vi "Start Arrival Time Counters TIO.vi"(7 "Save Data":bool, 8 "error in":errorcluster) -> (0 "error out":errorcluster, 1 "Column Definitions":T2(array[cluster]) {"Offset" format="%.2f"; "Resolution" format="%.2f"}, 2 "Buffer":i32[][](array[numeric]), 3 "Arrival Time Clusters":T3(array[cluster]), 5 "Temp File Definition":T1)   [LabVIEW 2009]
uses:
  Acquisition Settings.vi
panel:
  in  "Arrival Time Cluster":T4 {"task ID out" format="%.0x"}
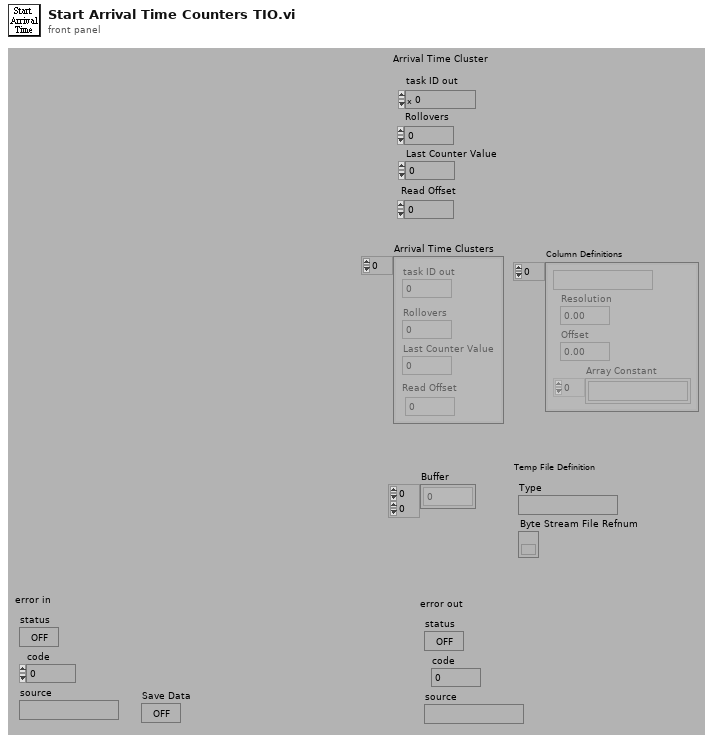
[diagram p1: front panel]
types:
  T1 = cluster{"Type":string, "Byte Stream File Refnum":refnum<file>}
  T2 = cluster{string, "Resolution":dbl, "Offset":dbl, "Array Constant":string[]}[]
  T3 = cluster{"task ID out":u32, "Rollovers":i32, "Last Counter Value":u32, "Read Offset":i32}[]
  T4 = cluster{"task ID out":u32, "Rollovers":i32, "Last Counter Value":u32, "Read Offset":i32}
  T5 = cluster{"Name":string, "Device Number":i16, "Counter Number":i16, "Line Type for Gate":u32, "Line Number for Gate":u32, "Line Type for Source":u32, "Line Number for Source":u32, "Transfer Method":u32, "Signal Routing Configuration":i16}[]
  T6 = cluster{string, dbl, "Offset":dbl, "Array Constant":string[]}
  T7 = cluster{string, "Resolution":dbl, "Offset":dbl, "Array Constant":string[]}
  T8 = cluster{"Name":string, "Signal Routing":cluster{"signal name":u16, "signal source":u16, "signal source line number":u32, "signal name line number":u32}[]}[]
  T9 = cluster{"Name":string, "Signal Routing":cluster{"signal name":u16, "signal source":u16, "signal source line number":u32, "signal name line number":u32}[]}
  T10 = cluster{"signal name":u16, "signal source":u16, "signal source line number":u32, "signal name line number":u32}[]
  T11 = cluster{string, "Offset":dbl, "Offset":dbl, string[]}
  T12 = cluster{string, "Offset":dbl, "Offset":dbl, "Array Constant":string[]}[]
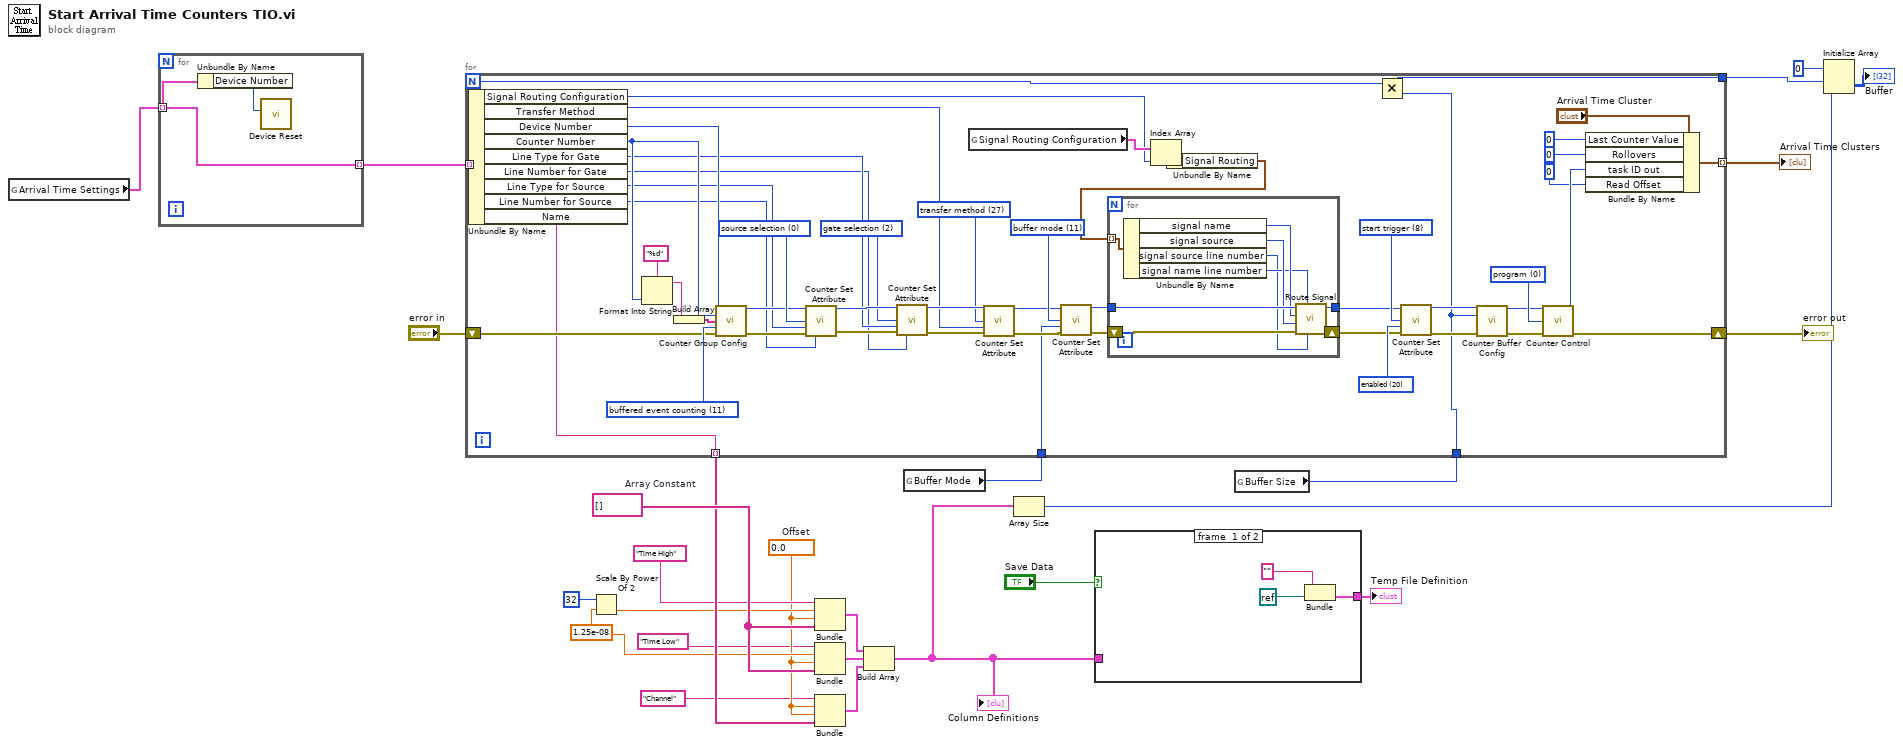
[diagram p0: block diagram]
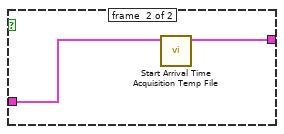
[diagram p2: hidden frame]
diagram:
  w9 = 0.0  # Offset
  w10 = 1.25e-08 ("Resolution")
  w18 = string[] []  # Array Constant
  n1 = global read "Acquisition Settings.vi" "Arrival Time Settings"() -> (w3:T5)
  n2 = for {
    tunnel: w3 -> [w28] mode=indexing
    tunnel: [w28] -> w4 mode=indexing
    n3 = Unbundle By Name(w28) -> ("Device Number"=w27:i16)
    n4 = call <vilib>:"Device Reset.vi"("device"=w27) -> ()  [unwired: 9 in, 2 out]
  }
  n5 = Scale By Power Of 2(n=32, x=w10) -> (x*2^n=w12:dbl)
  n6 = Bundle("Time High", w12, "Offset"=w9, "Array Constant"=w18) -> (w16:T6)  [unwired: 1 in]
  n7 = Bundle("Time Low", "Resolution"=w10, "Offset"=w9, "Array Constant"=w18) -> (w15:T7)  [unwired: 1 in]
  n8 = global read "Acquisition Settings.vi" "Buffer Mode"() -> (w2:u32)
  n9 = global read "Acquisition Settings.vi" "Buffer Size"() -> (w1:i32)
  n10 = for {
    N -> [w48]
    shift-right: [w60] -> w26
    shift-left: "error in" -> [w59]
    tunnel: w4 -> [w58] mode=indexing
    tunnel: [w47] -> w23
    tunnel: [w53] -> w22 mode=indexing
    tunnel: [w45] -> w17 mode=indexing
    tunnel: w2 -> [w38]
    tunnel: w1 -> [w37]
    w40 = u32 27 items=["source selection", "source polarity", "gate selection", "gate polarity", "output mode", "output polarity", "aux line selection", "aux line polarity", "start trigger", "counting synchronous", "up down", "buffer mode", "encoder type", "initial count", "pulse spec 1", "pulse spec 2", "pulse spec 3", "pulse spec 4", "auto increment", "prescale value", "Z index active", "Z index value", "Z index reload phase", "(Reserved) synchronization line", "(Reserved) synchronization method", "(Reserved) seconds", "(Reserved) precision", "transfer method", "start trigger polarity"] ("attribute ID")
    w54 = u32 20 items=["yes", "no", "positive", "negative", "high", "low", "low to high", "high to low", "default", "max timebase", "other counter gate", "other counter TC", "other counter output", "other counter source", "source", "gate", "aux line", "in start trigger", "in stop trigger", "automatic", "enabled", "count up", "count down", "hardware", "single", "double", "pulse", "toggle", "quadrature encoder X1", "quadrature encoder X2", "quadrature encoder X4", "two pulse counting", "A high B high", "A high B low", "A low B high", "A low B low", "PFI n", "RTSI n", "timebase n"] ("attribute value type")
    w55 = u32 8 items=["source selection", "source polarity", "gate selection", "gate polarity", "output mode", "output polarity", "aux line selection", "aux line polarity", "start trigger", "counting synchronous", "up down", "buffer mode", "encoder type", "initial count", "pulse spec 1", "pulse spec 2", "pulse spec 3", "pulse spec 4", "auto increment", "prescale value", "Z index active", "Z index value"] ("attribute ID")
    w65 = u32 11 items=["simple event counting", "single period measurement", "single pulse width measurement", "triggered pulse width measurement", "two signal edge separation measurement", "position measurement", "single pulse generation", "single triggered pulse generation", "retriggerable pulse generation", "pulse train generation", "frequency shift keying", "buffered event counting", "buffered period measurement", "buffered semiperiod measurement", "buffered pulse width measurement", "buffered two signal edge separation measurement", "buffered position measurement"] ("task type")
    w71 = u32 0 items=["source selection", "source polarity", "gate selection", "gate polarity", "output mode", "output polarity", "aux line selection", "aux line polarity", "start trigger", "counting synchronous", "up down", "buffer mode", "encoder type", "initial count", "pulse spec 1", "pulse spec 2", "pulse spec 3", "pulse spec 4", "auto increment", "prescale value", "Z index active", "Z index value"] ("attribute ID")
    w72 = u32 2 items=["source selection", "source polarity", "gate selection", "gate polarity", "output mode", "output polarity", "aux line selection", "aux line polarity", "start trigger", "counting synchronous", "up down", "buffer mode", "encoder type", "initial count", "pulse spec 1", "pulse spec 2", "pulse spec 3", "pulse spec 4", "auto increment", "prescale value", "Z index active", "Z index value"] ("attribute ID")
    w75 = u32 11 items=["source selection", "source polarity", "gate selection", "gate polarity", "output mode", "output polarity", "aux line selection", "aux line polarity", "start trigger", "counting synchronous", "up down", "buffer mode", "encoder type", "initial count", "pulse spec 1", "pulse spec 2", "pulse spec 3", "pulse spec 4", "auto increment", "prescale value", "Z index active", "Z index value"] ("attribute ID")
    w80 = u32 0 items=["program", "reset", "arm", "prepare", "disarm", "count up", "count down", "switch cycle", "snapshot"] ("control code")
    n11 = Unbundle By Name(w58) -> ("Signal Routing Configuration"=w29:i16, "Transfer Method"=w39:u32, "Device Number"=w76:i16, "Counter Number"=w77:i16, "Line Type for Gate"=w64:u32, "Line Number for Gate"=w63:u32, "Line Type for Source"=w62:u32, "Line Number for Source"=w61:u32, "Name"=w45:string)
    n12 = Format Into String(format string="%d" ("Format String"), w77) -> (resulting string=w67:string)  [unwired: 2 in, 1 out]
    n13 = Build Array(w67) -> (w68:string[])
    n14 = call <vilib>:"Counter Group Config.vi"("device"=w76, "group"=w77, "counter list"=w68, "task type"=w65, "error in (no error)"=w59) -> ("task ID"=w70:u32, "error out"=w69:errorcluster)  [unwired: 8 in, 1 out]
    n15 = call <vilib>:"Counter Set Attribute.vi"("task ID in"=w70, "attribute ID"=w71, "attribute value type"=w62, "error in (no error)"=w69, "attribute value number"=w61) -> ("task ID out"=w73:u32, "error out"=w74:errorcluster)  [unwired: 9 in]
    n16 = call <vilib>:"Counter Set Attribute.vi"("task ID in"=w73, "attribute ID"=w72, "attribute value type"=w64, "error in (no error)"=w74, "attribute value number"=w63) -> ("task ID out"=w44:u32, "error out"=w42:errorcluster)  [unwired: 9 in]
    n17 = global read "Acquisition Settings.vi" "Signal Routing Configuration"() -> (w30:T8)
    n18 = call <vilib>:"Counter Set Attribute.vi"("task ID in"=w44, "attribute ID"=w40, "attribute value type"=w39, "error in (no error)"=w42) -> ("task ID out"=w43:u32, "error out"=w41:errorcluster)  [unwired: 10 in]
    n19 = call <vilib>:"Counter Set Attribute.vi"("task ID in"=w43, "attribute ID"=w75, "attribute value type"=w38, "error in (no error)"=w41) -> ("task ID out"=w34:u32, "error out"=w33:errorcluster)  [unwired: 10 in]
    n20 = Index Array(array=w30, index=w29) -> (element=w35:T9)
    n21 = Unbundle By Name(w35) -> ("Signal Routing"=w36:T10)
    n22 = for {
      tunnel: w34 -> [w89]
      shift-right: [w81] -> w32
      shift-left: w33 -> [w88]
      tunnel: w36 -> [w87] mode=indexing
      tunnel: [w82] -> w31
      n23 = Unbundle By Name(w87) -> ("signal name"=w86:u16, "signal source"=w85:u16, "signal source line number"=w83:u32, "signal name line number"=w84:u32)
      n24 = call <vilib>:"Route Signal.vi"("signal source line number"=w83, "signal name line number"=w84, "error in (no error)"=w88, "signal source"=w85, "signal name"=w86, "task ID"=w89) -> ("error out"=w81:errorcluster, "task ID out"=w82:u32)  [unwired: 4 in]
    }
    n25 = Multiply(x=w48, y=w37) -> (x*y=w47:i32)
    n26 = call <vilib>:"Counter Set Attribute.vi"("task ID in"=w31, "attribute ID"=w55, "attribute value type"=w54, "error in (no error)"=w32) -> ("task ID out"=w57:u32, "error out"=w56:errorcluster)  [unwired: 10 in]
    n27 = call <vilib>:"Counter Buffer Config.vi"("task ID in"=w57, "counts per buffer"=w37, "error in (no error)"=w56) -> ("task ID out"=w78:u32, "error out"=w79:errorcluster)  [unwired: 11 in]
    n28 = call <vilib>:"Counter Control.vi"("task ID"=w78, "control code"=w80, "error in (no error)"=w79) -> ("task ID out"=w51:u32, "error out"=w60:errorcluster)  [unwired: 11 in]
    n29 = Bundle By Name(cluster="Arrival Time Cluster", "Last Counter Value"=u32 0 ("Bundle Element"), "Rollovers"=0 ("Bundle Element"), "task ID out"=w51, "Read Offset"=0 ("Bundle Element")) -> (w53:T4)
  }
  "error out" <- w26
  "Arrival Time Clusters" <- w22
  n30 = Bundle("Channel", "Offset"=w9, "Offset"=w9, w17) -> (w14:T11)  [unwired: 1 in]
  n31 = Build Array(w16, w15, w14) -> (w6:T12)
  "Column Definitions" <- w6
  n32 = Array Size(array=w6) -> (size(s)=w19:i32)
  n33 = case shown="True" "Save Data" {
    tunnel: [w90 w94] -> w5
    tunnel: w6 -> [_ w93]
    frame #0 {
      n34 = Bundle("", refnum<k0> refnum) -> (w90:cluster{string, refnum<k0>})  [unwired: 1 in]
    }
    frame #1 {
      n35 = call "Start Arrival Time Acquisition Temp File.vi"("Column Definitions"=w93) -> ("Temp File Definition"=w94:T1)  [unwired: 9 in, 1 out]
    }
  }
  "Temp File Definition" <- w5
  n36 = Initialize Array(0 ("Element Data"), w23, w19) -> (→"Buffer":i32[][])
